vi "SamplingRate.vi"() -> ()   [LabVIEW 2016]
uses:
  <vilib>/LabVIEW Interface for Arduino/Type Defs/Arduino Resource.ctl
  <vilib>/LabVIEW Interface for Arduino/Type Defs/Board Type.ctl
  <vilib>/LabVIEW Interface for Arduino/Type Defs/Pin Mode.ctl
  <vilib>/LabVIEW Interface for Arduino/LabVIEW Interface for Arduino.lvlib
panel:
  out "Trial No.":i32
  in  "Cycle Time [ms]":dbl=10000.0 format="%#_13g"
  in  "Pulse Length [ms]":dbl=125.0 format="%#_13g"
  in  "Iterations":i32=20
  out "Arduino Resource":T1={"VISA resource"="GlueCTRL", "Board Type"=enum."Uno", "Connection Type"=enum."USB / Serial", "Bytes Per Packet (15)"=15}
  in  "Digital I/O Pin":u8=7
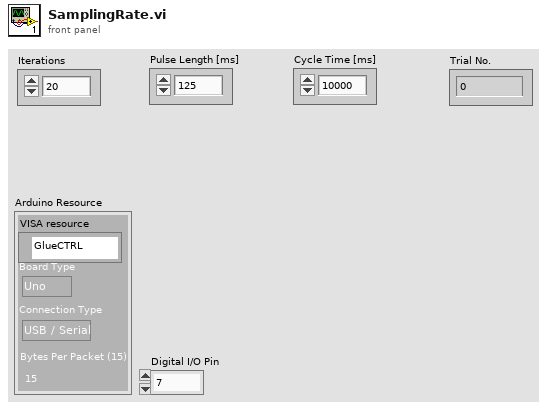
[diagram p1: front panel]
types:
  T1 = typedef "LabVIEW Interface for Arduino.lvlib/Arduino Resource.ctl" = cluster{"VISA resource":refnum<visa-resource-name>, "Board Type":T2, "Connection Type":enum8{"USB / Serial"}, "Bytes Per Packet (15)":u8}
  T2 = typedef "LabVIEW Interface for Arduino.lvlib/Board Type.ctl" = enum16{"Uno", "Dimuelanove w/Atmega 328", "Mega 2560"}
  T3 = typedef "LabVIEW Interface for Arduino.lvlib/Pin Mode.ctl" = enum8{"Input", "Output"}
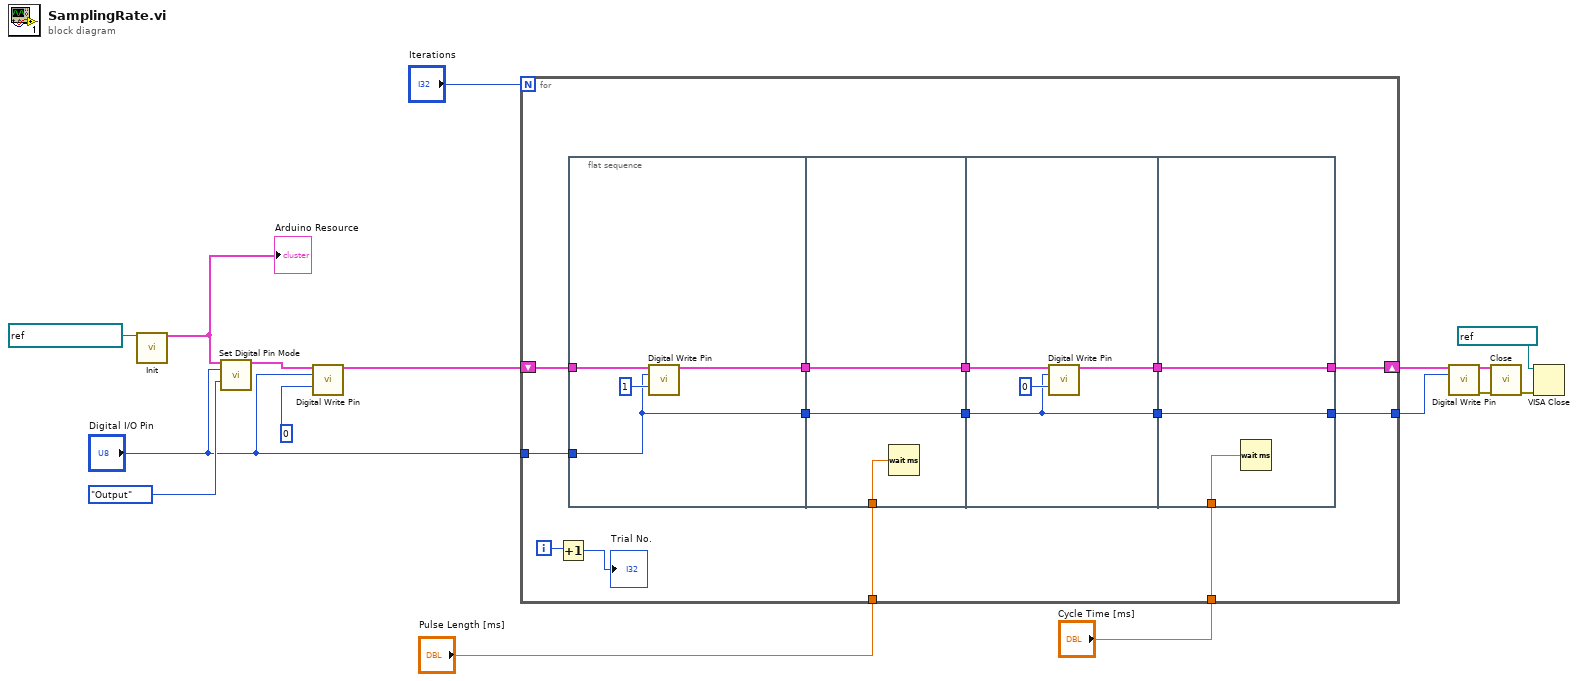
[diagram p0: block diagram]
diagram:
  n1 = call <vilib>:"Init.vi"("VISA resource"=refnum<visa-resource-name> "GlueCTRL") -> ("Arduino Resource"=w12:T1)  [unwired: 17 in, 1 out]
  "Arduino Resource" <- w12
  n2 = call <vilib>:"Set Digital Pin Mode.vi"("Arduino Resource"=w12, "Digital I/O Pin"="Digital I/O Pin", "Pin Mode (Input)"=Pin_Mode."Output") -> ("Arduino Resource"=w14:T1)  [unwired: 11 in, 1 out]
  n3 = call <vilib>:"Digital Write Pin.vi"("Arduino Resource"=w14, "Digital I/O Pin (0)"="Digital I/O Pin", "Value (0)"=u8 0) -> ("Arduino Resource"=w9:T1)  [unwired: 11 in, 1 out]
  n4 = for {
    N: "Iterations" -> [_]
    tunnel: "Digital I/O Pin" -> [w29]
    tunnel: "Pulse Length [ms]" -> [w28]
    tunnel: [w22] -> w2
    shift-right: [w23] -> w3
    shift-left: w9 -> [w30]
    tunnel: "Cycle Time [ms]" -> [w19]
    i -> [w18]
    n5 = Increment(x=w18) -> (x+1=→"Trial No.":i32)
    n6 = flat-sequence {
      tunnel: w30 -> [w33]
      tunnel: w29 -> [w31]
      tunnel: [w32] -> w26
      tunnel: [w31] -> w24
      tunnel: w28 -> [w37]
      tunnel: [w36] -> w27
      tunnel: w26 -> [w36]
      tunnel: [w35] -> w25
      tunnel: w24 -> [w35]
      tunnel: w27 -> [w40]
      tunnel: w25 -> [w38]
      tunnel: [w39] -> w21
      tunnel: [w38] -> w20
      tunnel: [w43] -> w22
      tunnel: [w44] -> w23
      tunnel: w21 -> [w44]
      tunnel: w20 -> [w43]
      tunnel: w19 -> [w42]
      frame #0 {
        n7 = call <vilib>:"Digital Write Pin.vi"("Arduino Resource"=w33, "Digital I/O Pin (0)"=w31, "Value (0)"=u8 1) -> ("Arduino Resource"=w32:T1)  [unwired: 11 in, 1 out]
      }
      frame #1 {
        n8 = Wait (ms)(milliseconds to wait=w37) -> ()  [unwired: 1 out]
      }
      frame #2 {
        n9 = call <vilib>:"Digital Write Pin.vi"("Arduino Resource"=w40, "Digital I/O Pin (0)"=w38, "Value (0)"=u8 0) -> ("Arduino Resource"=w39:T1)  [unwired: 11 in, 1 out]
      }
      frame #3 {
        n10 = Wait (ms)(milliseconds to wait=w42) -> ()  [unwired: 1 out]
      }
    }
  }
  n11 = call <vilib>:"Digital Write Pin.vi"("Arduino Resource"=w3, "Digital I/O Pin (0)"=w2) -> ("Arduino Resource"=w6:T1, "error out"=w5:errorcluster)  [unwired: 12 in]
  n12 = call <vilib>:"Close.vi"("Arduino Resource"=w6, "error in"=w5) -> ("error out"=w4:errorcluster)  [unwired: 13 in]
  n13 = VISA Close(VISA resource name=refnum<visa-resource-name> "GlueCTRL", error in (no error)=w4) -> ()  [unwired: 1 out]
